vi "UN_PSWRD_2.0.vi"() -> ()   [LabVIEW 2019]
panel:
  in  "PASSWORD 2":string
  in  "USERNAME 2":string
  in  "Password_List":string[](array[string])
  in  "Username_list":string[](array[string])
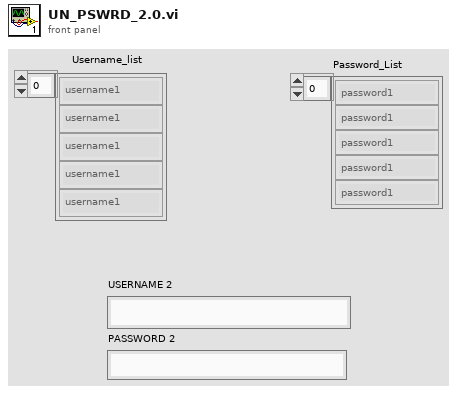
[diagram p1: front panel]
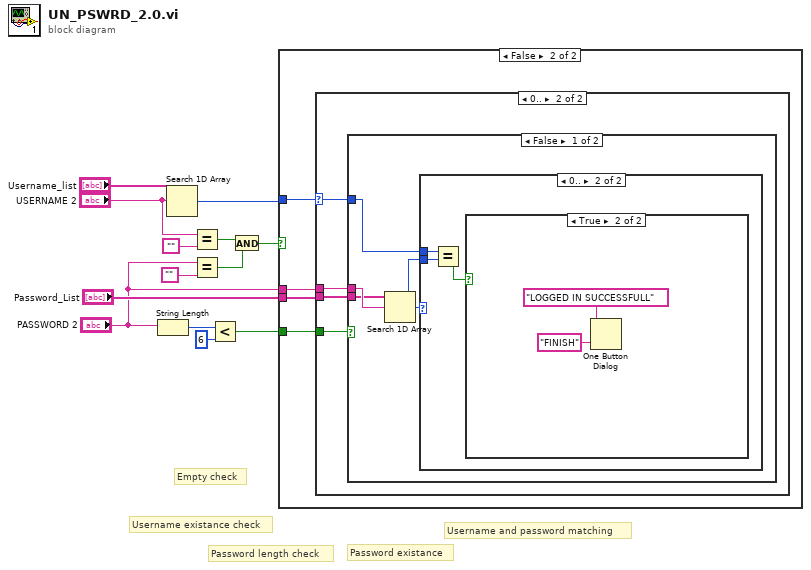
[diagram p0: block diagram]
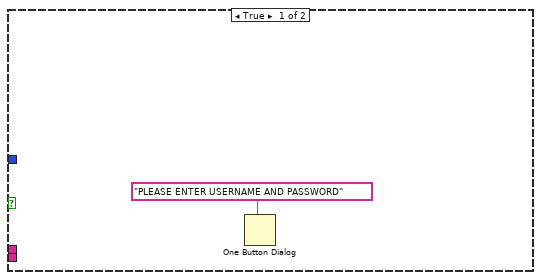
[diagram p2: hidden frame]
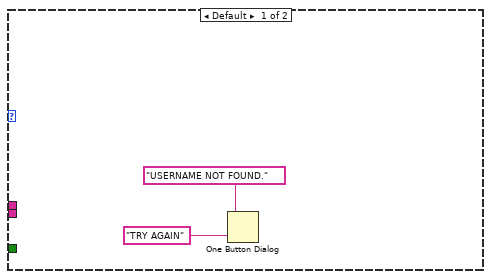
[diagram p3: hidden frame]
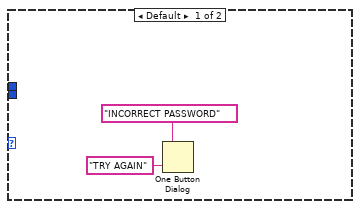
[diagram p4: hidden frame]
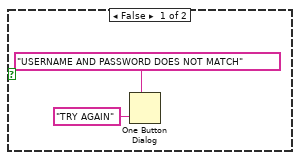
[diagram p5: hidden frame]
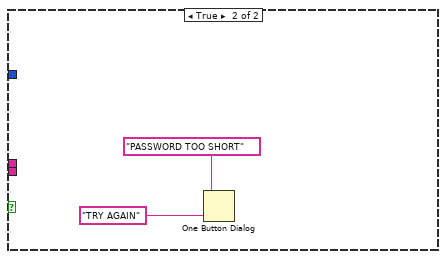
[diagram p6: hidden frame]
diagram:
  # "Username and password matching"
  # "Password existance"
  # "Password length check"
  # "Username existance check"
  # "Empty check"
  n1 = String Length(string="PASSWORD 2") -> (length=w12:i32)
  n2 = Search 1D Array(1D array="Username_list", element="USERNAME 2") -> (index of element=w10:i32)  [unwired: 1 in]
  n3 = Equal?(x="USERNAME 2", y="") -> (x = y?=w2:bool)
  n4 = Equal?(x="PASSWORD 2", y="") -> (x = y?=w3:bool)
  n5 = Less?(x=w12, y=6) -> (x < y?=w9:bool)
  n6 = And(x=w2, y=w3) -> (x .and. y?=w1:bool)
  n7 = case shown="False" w1 {
    tunnel: w10 -> [_ w18]
    tunnel: w9 -> [_ w17]
    tunnel: "PASSWORD 2" -> [_ w16]
    tunnel: "Password_List" -> [_ w15]
    frame True {
      n8 = One Button Dialog(message="PLEASE ENTER USERNAME AND PASSWORD") -> ()  [unwired: 1 in, 1 out]
    }
    frame False {
      n9 = case shown="0.." w18 {
        selector: w18 -> [_ w21]
        tunnel: w17 -> [_ w24]
        tunnel: w16 -> [_ w23]
        tunnel: w15 -> [_ w22]
        frame Default {
          n10 = One Button Dialog(message="USERNAME NOT FOUND.", button name ("OK")="TRY AGAIN") -> ()  [unwired: 1 out]
        }
        frame 0.. {
          n11 = case shown="False" w24 {
            tunnel: w23 -> [w28 _]
            tunnel: w22 -> [w27 _]
            tunnel: w21 -> [w26 _]
            frame False {
              n12 = Search 1D Array(1D array=w27, element=w28) -> (index of element=w25:i32)  [unwired: 1 in]
              n13 = case shown="0.." w25 {
                tunnel: w26 -> [_ w33]
                tunnel: w25 -> [_ w31]
                frame Default {
                  n14 = One Button Dialog(message="INCORRECT PASSWORD", button name ("OK")="TRY AGAIN") -> ()  [unwired: 1 out]
                }
                frame 0.. {
                  n15 = Equal?(x=w33, y=w31) -> (x = y?=w32:bool)
                  n16 = case shown="True" w32 {
                    frame False {
                      n17 = One Button Dialog(message="USERNAME AND PASSWORD DOES NOT MATCH", button name ("OK")="TRY AGAIN") -> ()  [unwired: 1 out]
                    }
                    frame True {
                      n18 = One Button Dialog(message="LOGGED IN SUCCESSFULL", button name ("OK")="FINISH") -> ()  [unwired: 1 out]
                    }
                  }
                }
              }
            }
            frame True {
              n19 = One Button Dialog(message="PASSWORD TOO SHORT", button name ("OK")="TRY AGAIN") -> ()  [unwired: 1 out]
            }
          }
        }
      }
    }
  }
